vi "startup.vi"(8 "error in (no error)":errorcluster, 11 "ActionEditor in":refnum<class "ActionEditor.lvclass">) -> (0 "error out":errorcluster, 3 "ActionEditor out":refnum<class "ActionEditor.lvclass">)   [LabVIEW 2009, in "Views.lvlib" / "ScriptEditor.lvlib" / "ActionEditor.lvclass"]
uses:
  ActionEditor.lvclass
  ActionEditor.lvclass/ActionEditor.ctl
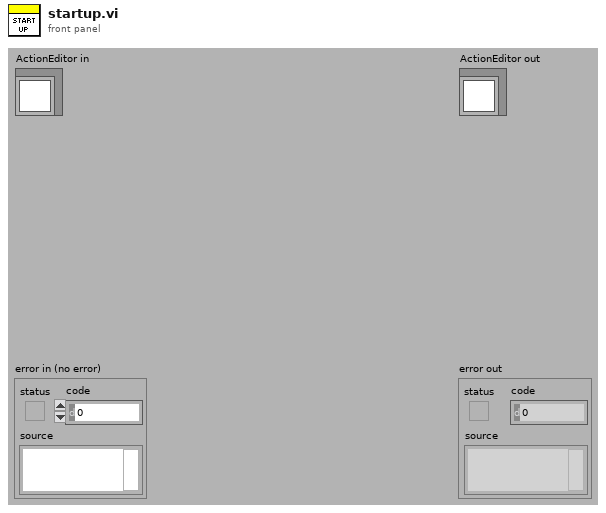
[diagram p1: front panel]
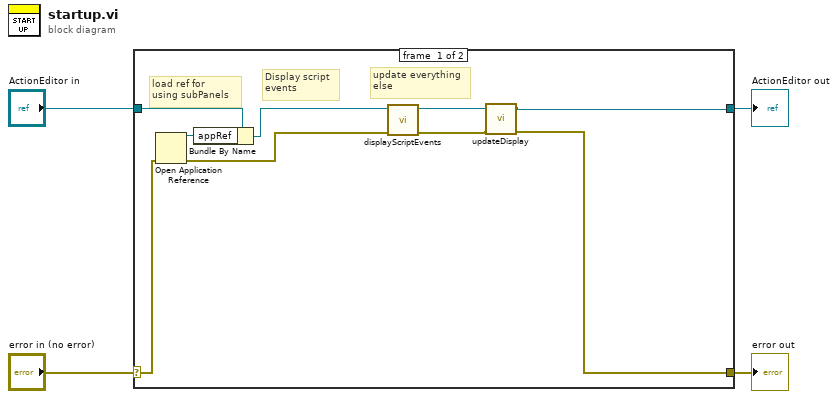
[diagram p0: block diagram]
diagram:
  n1 = case shown="No Error" "error in (no error)" {
    selector: "error in (no error)" -> [w11 w15]
    tunnel: [w5 w15] -> w3
    tunnel: [w6 w14] -> w1
    tunnel: "ActionEditor in" -> [w13 w14]
    frame #0 {
      # "update everything\nelse"
      # "Display script \nevents"
      # "load ref for\nusing subPanels"
      n2 = Open Application Reference(8:w11) -> (0:w9:errorcluster, 3:w12:refnum<vi>)  [unwired: 3 in]
      n3 = Bundle By Name(cluster=w13, "appRef"=w12) -> (w10:refnum<class "ActionEditor.lvclass">)
      n4 = call "displayScriptEvents.vi"("error in (no error)"=w9, "ActionEditor in"=w10) -> ("error out"=w7:errorcluster, "ActionEditor out"=w8:refnum<class "ActionEditor.lvclass">)  [unwired: 8 in]
      n5 = call "updateDisplay.vi"("error in (no error)"=w7, "ActionEditor in"=w8) -> ("error out"=w5:errorcluster, "ActionEditor out"=w6:refnum<class "ActionEditor.lvclass">)  [unwired: 8 in]
    }
    frame #1 {
    }
  }
  "error out" <- w3
  "ActionEditor out" <- w1
